vi "Set Fast Kinetics Ex.vi"(4 "offset":i32, 5 "vbin":i32, 6 "hbin":i32, 7 "mode":i32, 8 "error in (no error)":errorcluster, 9 "time":sgl, 10 "seriesLength":i32, 11 "exposedRows":i32) -> (0 "error out":errorcluster, 3 "function return":u32)   [LabVIEW 2014, in "atmcd32d.lvlib"]
doc: "unsigned int WINAPI SetFastKineticsEx(int exposedRows, int seriesLength, float time, int mode, int hbin, int vbin, int offset);"
uses:
  atmcd32d.lvlib
  atmcd32d.dll
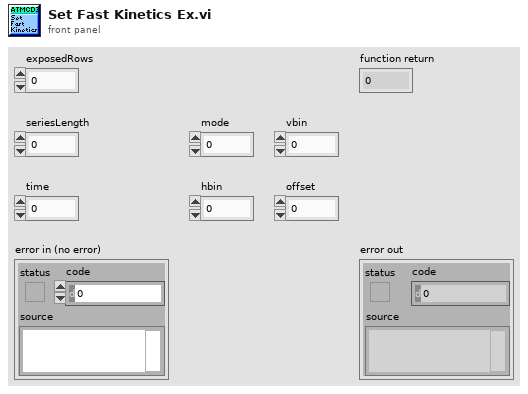
[diagram p1: front panel]
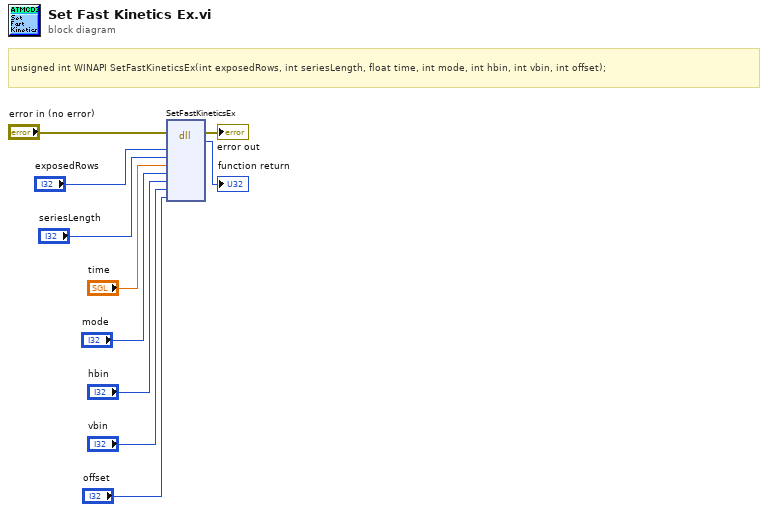
[diagram p0: block diagram]
diagram:
  # "unsigned int WINAPI SetFastKineticsEx(int exposedRows, int seriesLength, float time, int mode, int hbin, int vbin, int offset);"
  n1 = dll-call lib="C:/Users/Bakir/Documents/Lambda2-Testing/lib/Andorlib/atmcd32d.*" fn="SetFastKineticsEx"(error in="error in (no error)", "exposedRows"="exposedRows", "seriesLength"="seriesLength", "time"="time", "mode"="mode", "hbin"="hbin", "vbin"="vbin", "offset"="offset") -> (error out=→"error out":errorcluster, →"function return":u32)  [unwired: 9 in, 1 out]
